vi "Open VI FP.vi"(8 "error in (no error)":errorcluster, 11 "VIPath":path) -> (0 "error out":errorcluster)   [LabVIEW 2014]
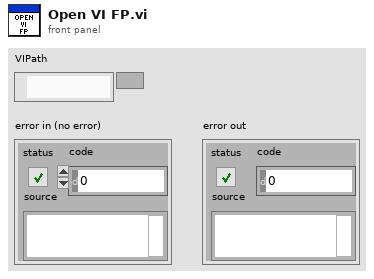
[diagram p1: front panel]
types:
  T1 = enum32{"Invalid", "Standard", "Closed", "Hidden", "Minimized", "Maximized"}
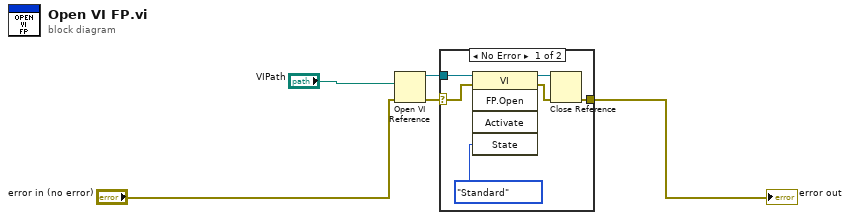
[diagram p0: block diagram]
diagram:
  n1 = Open VI Reference(vi path="VIPath", error in (no error)="error in (no error)") -> (vi reference=w1:refnum<vi>, error out=w2:errorcluster)  [unwired: 4 in]
  n2 = case shown="No Error" w2 {
    selector: w2 -> [w10 w12]
    tunnel: w1 -> [w11 _]
    tunnel: [w6 w12] -> w4
    frame No Error {
      n3 = invoke class="VI" method="FP.Open"(reference=w11, error in=w10, "State"=T1."Standard") -> (reference out=w8:refnum<vi>, error out=w9:errorcluster)  [unwired: 2 in, 3 out]
      n4 = Close Reference(reference=w8, error in (no error)=w9) -> (error out=w6:errorcluster)
    }
    frame Error {
    }
  }
  "error out" <- w4
